vi "Update.vi"(8 "error in (no error)":errorcluster, 10 "enable":bool=TRUE) -> (0 "error out":errorcluster)   [LabVIEW 2017, in "RTProtocol.lvlib"]
uses:
  <vilib>/addons/InsightCM/Utilities/Security/RTProtocol/RTProtocol.lvlib
  <vilib>/Utility/config.llb/Write Key (Boolean).vi
  <vilib>/Utility/config.llb/NI_LVConfig.lvlib
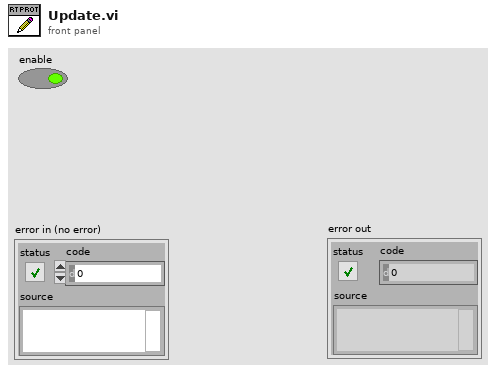
[diagram p1: front panel]
types:
  T1 = typedef "NI_LVConfig.lvlib/Config Data RefNum.ctl" = refnum<k1>
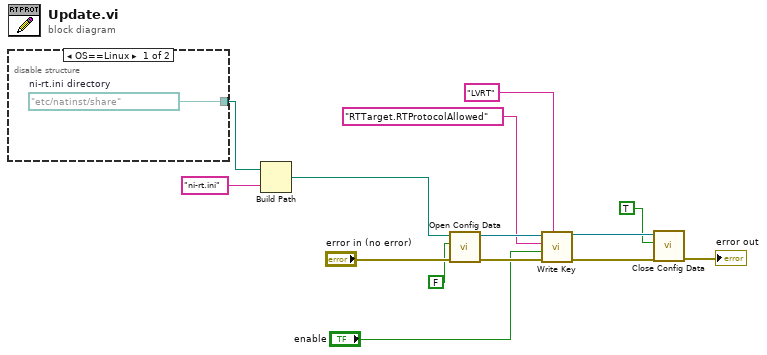
[diagram p0: block diagram]
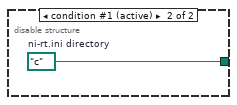
[diagram p2: hidden frame]
diagram:
  n1 = disable-structure shown="OS==Linux" {
    disable-tunnel: [w15 w16] -> w2
    frame condition #0 {
      w15 = path "/etc/natinst/share"  # ni-rt.ini directory
    }
    frame condition #1 (active) {
      w16 = path "c:/"  # ni-rt.ini directory
    }
  }
  n2 = Build Path(base path=w2, name or relative path="ni-rt.ini") -> (appended path=w4:path)
  n3 = call <vilib>:"Open Config Data.vi"("error in (no error)"="error in (no error)", "create file if necessary (T)"=FALSE, "configuration file path"=w4) -> ("error out"=w13:errorcluster, "refnum"=w10:T1)  [unwired: 6 in, 1 out]
  n4 = call-poly <vilib>:"Write Key.vi"("section"="LVRT", "error in (no error)"=w13, "value"="enable", "key"="RTTarget.RTProtocolAllowed", "refnum"=w10) -> ("error out"=w12:errorcluster, "refnum out"=w11:T1)  [unwired: 4 in, 1 out]
  n5 = call <vilib>:"Close Config Data.vi"("error in (no error)"=w12, "write file if changed (T)"=TRUE, "refnum"=w11) -> ("error out"=→"error out":errorcluster)  [unwired: 7 in, 1 out]
